vi "Finalize.vi"(8 "error in":errorcluster, 11 "Plugin in":refnum<class "Sequencer with Output Values.lvclass">) -> (0 "error out":errorcluster, 3 "Plugin out":refnum<class "Sequencer with Output Values.lvclass">)   [LabVIEW 2024, in "Sequencer with Output Values.lvlib" / "Sequencer with Output Values.lvclass"]
uses:
  Sequencer with Output Values.lvclass
  C:/Program Files/National Instruments/LabVIEW 2024/vi.lib/FlexLogger/SDK/PluginSDK.lvlibp/PEFClasses/SDK/Processing Element/Processing Element.lvclass
  Tree Manager/Tree Manager Mode.ctl
  Sequencer with Output Values.lvclass/Sequencer with Output Values.ctl
  <vilib>/FlexLogger/SDK/PluginSDK.lvlibp/PEFClasses/SDK/Processing Element/Read Alias.vi
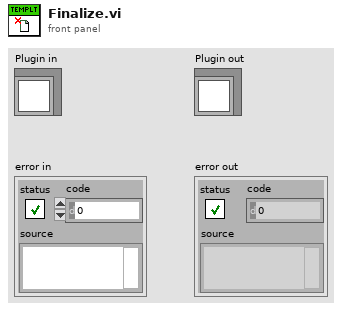
[diagram p1: front panel]
types:
  T1 = typedef "Sequencer with Output Values.lvlib/Sequencer with Output Values.lvclass/Tree Manager Mode.ctl" = enum16{"Init", "Tree Change", "Value Change", "Close"}
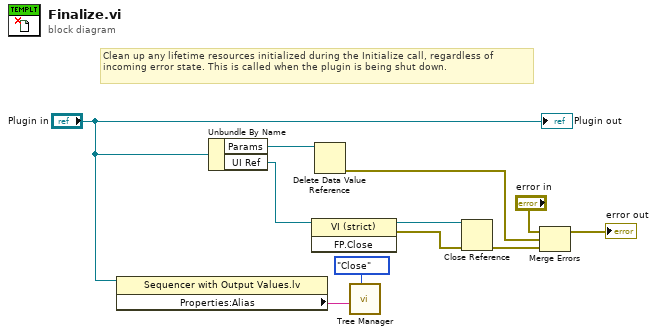
[diagram p0: block diagram]
diagram:
  # "Clean up any lifetime resources initialized during the Initialize call, regardless of incoming error state. This is called when the plugin is being shut down."
  n1 = property class="Sequencer with Output Values.lv"(reference="Plugin in") -> ("Properties:Alias"=w1:string)  [unwired: 1 in, 2 out]
  n2 = Unbundle By Name("Plugin in") -> ("Params"=w10:refnum<data-value>, "UI Ref"=w6:refnum<vi>)
  n3 = invoke class="VI (strict)" method="FP.Close"(reference=w6) -> (reference out=w5:refnum<vi>, error out=w4:errorcluster)  [unwired: 2 in, 1 out]
  n4 = Delete Data Value Reference(data value reference=w10) -> (error out=w9:errorcluster)  [unwired: 1 in, 1 out]
  n5 = call "Tree Manager.vi"("Mode"=Tree_Manager_Mode."Close", "Alias"=w1) -> ()  [unwired: 9 in, 1 out]
  n6 = Close Reference(reference=w5, error in (no error)=w4) -> (error out=w8:errorcluster)
  n7 = Merge Errors("error in", w9, w8) -> (→"error out":errorcluster)
  "Plugin out" <- "Plugin in"
